vi "toml_fg.vi"(5 "action":T1, 6 "comment in":string, 7 "section":string[](array[string]), 8 "error in (no error)":errorcluster, 9 "value in":string, 10 "key":string[](array[string]), 11 "path in":path) -> (0 "error out":errorcluster, 1 "value out":string, 2 "exists?":bool, 3 "path out":path, 4 "comment out":string)   [LabVIEW 2017]
uses:
  toml_key_action.ctl
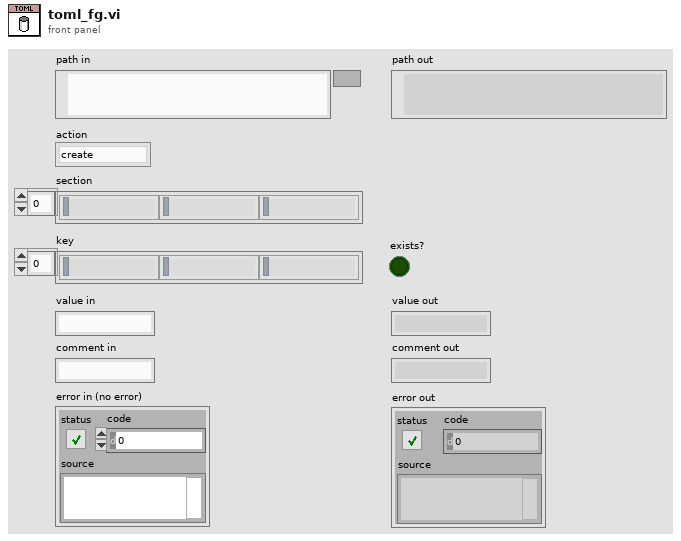
[diagram p1: front panel]
types:
  T1 = typedef "toml_key_action.ctl" = enum8{"create", "read", "write", "delete"}
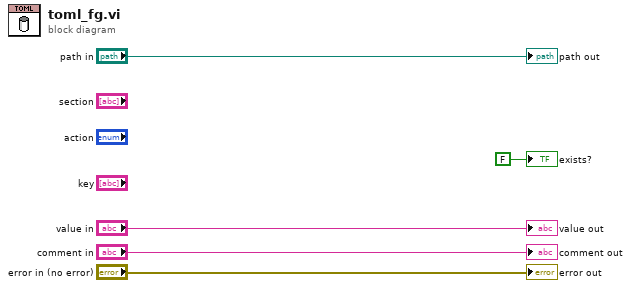
[diagram p0: block diagram]
diagram:
  "error out" <- "error in (no error)"
  "value out" <- "value in"
  "exists?" <- FALSE ("exists?")
  "path out" <- "path in"
  "comment out" <- "comment in"
